vi "Read Client types.vi"(8 "error in (no error)":errorcluster, 11 "Get-clients in":refnum<class "Get-clients.lvclass">) -> (0 "error out":errorcluster, 2 "Client types":string[](array[string]), 3 "Get-clients out":refnum<class "Get-clients.lvclass">)   [LabVIEW 2013, in "Messages.lvlib" / "Get-clients.lvclass"]
uses:
  Get-clients.lvclass
  Get-clients.lvclass/Get-clients.ctl
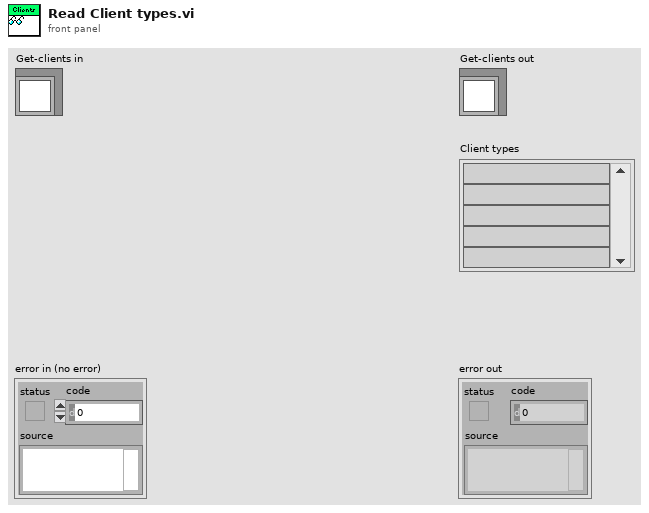
[diagram p1: front panel]
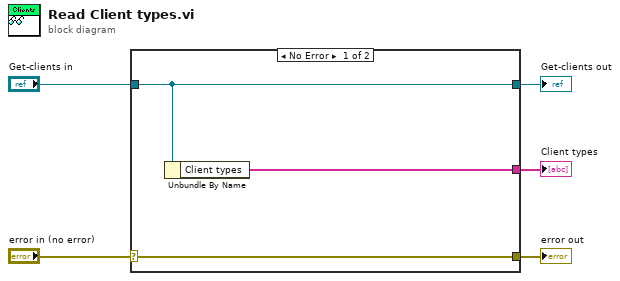
[diagram p0: block diagram]
diagram:
  n1 = case shown="No Error" "error in (no error)" {
    selector: "error in (no error)" -> [w8 w9]
    tunnel: [w8 w9] -> w4
    tunnel: [w7 w10] -> w2
    tunnel: "Get-clients in" -> [w7 w10]
    tunnel: [w6 _] -> w1
    frame No Error {
      n2 = Unbundle By Name(w7) -> ("Client types"=w6:string[])
    }
    frame Error {
    }
  }
  "error out" <- w4
  "Get-clients out" <- w2
  "Client types" <- w1
